vi "All UI States.vi"() -> (2 "All UI States":T1[](array[typedef]))   [LabVIEW 2022 SP3, in "FlexBlocks Support.lvlib"]
uses:
  FlexBlocks Support.lvlib
  UI State.ctl
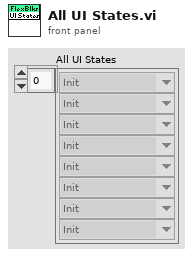
[diagram p1: front panel]
types:
  T1 = typedef "FlexBlocks Support.lvlib/UI State.ctl" = enum16{"Init", "Load", "Ready", "Run", "Cleanup", "Close"}
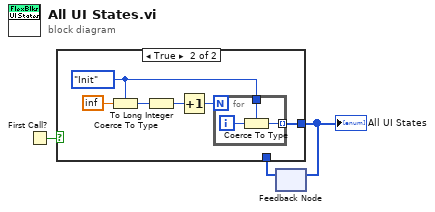
[diagram p0: block diagram]
diagram:
  n1 = First Call?() -> (First Call?: T/F=w1:bool)
  n2 = feedback #1() -> (w2:T1[])  [unwired: 1 in]
  n3 = case shown="True" w1 {
    tunnel: [w4 w6] -> w3
    tunnel: w2 -> [w4 _]
    frame False {
    }
    frame True {
      w7 = UI_State."Init" ("UI State")
      n4 = Coerce To Type(0:inf, 1:w7) -> (2:w9:T1)
      n5 = To Long Integer(number=w9) -> (32bit integer=w8:i32)
      n6 = Increment(x=w8) -> (x+1=w5:i32)
      n7 = for {
        N: w5 -> [_]
        tunnel: w7 -> [w12]
        tunnel: [w11] -> w6 mode=indexing
        i -> [w13]
        n8 = Coerce To Type(0:w13, 1:w12) -> (2:w11:T1)
      }
    }
  }
  "All UI States" <- w3
  n9 = feedback-in #1(w3) -> ()
